vi "build_digitimer_trigger.vi"(6 "Padding (ms)":dbl, 9 "Stim Duration (ms)":dbl, 10 "Sampling Freq (hz)":dbl, 11 "Stim Freq (hz)":dbl) -> (1 "waveform out":waveform(dbl), 2 "number of samples":i32, 3 "duration":dbl)   [LabVIEW 2020]
uses:
  <vilib>/measure/NI_MABase.lvlib
  <vilib>/Waveform/WDTOps.llb/WDT Append Waveforms DBL.vi
  <vilib>/Waveform/WDTOps.llb/WDT Waveform Duration DBL.vi
  <vilib>/Waveform/WDTOps.llb/WDT Number of Waveform Samples DBL.vi
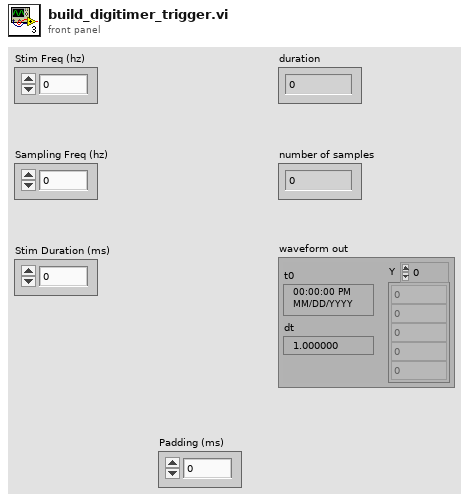
[diagram p1: front panel]
types:
  T1 = cluster{"Sampling Freq (hz)":dbl, "Stim Duration (ms)":dbl}
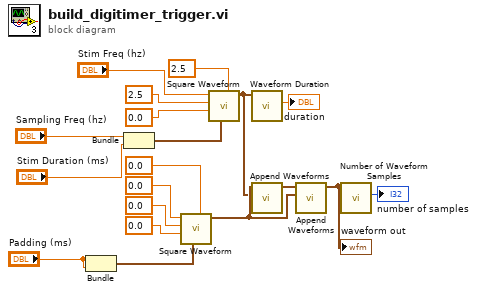
[diagram p0: block diagram]
diagram:
  n1 = Bundle("Padding (ms)"="Padding (ms)", "Padding (ms)"="Padding (ms)") -> (w18:cluster{"Padding (ms)":dbl, "Padding (ms)":dbl})  [unwired: 1 in]
  n2 = Bundle("Sampling Freq (hz)"="Sampling Freq (hz)", "Stim Duration (ms)"="Stim Duration (ms)") -> (w14:T1)  [unwired: 1 in]
  n3 = call <vilib>:"Square Waveform.vi"("offset"=0.0, "sampling info"=w18, "phase"=0.0 ("phase 2"), "amplitude"=0.0, "frequency"=0.0 ("frequency 2")) -> ("signal out"=w5:waveform(dbl))  [unwired: 5 in, 1 out]
  n4 = call <vilib>:"Square Waveform.vi"("offset"=2.5, "sampling info"=w14, "phase"=0.0, "amplitude"=2.5, "frequency"="Stim Freq (hz)") -> ("signal out"=w4:waveform(dbl))  [unwired: 5 in, 1 out]
  n5 = call-poly <vilib>:"Waveform Duration.vi"("waveform in"=w4) -> ("duration"=→"duration":dbl)  [unwired: 8 in, 2 out]
  n6 = call-poly <vilib>:"Append Waveforms.vi"("waveform B"=w4, "waveform A"=w5) -> ("waveform out"=w6:waveform(dbl))  [unwired: 8 in, 1 out]
  n7 = call-poly <vilib>:"Append Waveforms.vi"("waveform B"=w5, "waveform A"=w6) -> ("waveform out"=w2:waveform(dbl))  [unwired: 8 in, 1 out]
  "waveform out" <- w2
  n8 = call-poly <vilib>:"Number of Waveform Samples.vi"("waveform in"=w2) -> ("number of samples"=→"number of samples":i32)  [unwired: 8 in, 2 out]
